vi "Set Header and Data.vi"(6 "Data Array":dbl[](array[numeric]), 8 "error in (no error)":errorcluster, 9 "Data & Time String":string, 10 "Header":string, 11 "Report.lvclass in":refnum<class "Wind Report.lvclass">) -> (0 "error out":errorcluster, 3 "Report.lvclass out":refnum<class "Wind Report.lvclass">)   [LabVIEW 2009, in "Wind Report.lvclass"]
doc: "This parent method sets object data and can operate on the child object.\n\nAAL 9/09"
uses:
  Wind Report.lvclass
  Wind Report.lvclass/Wind Report.ctl
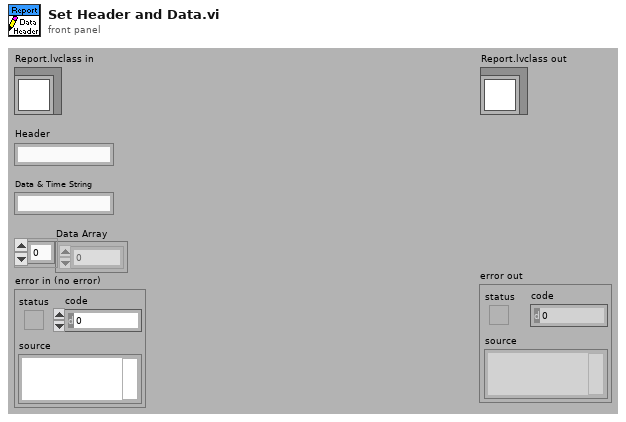
[diagram p1: front panel]
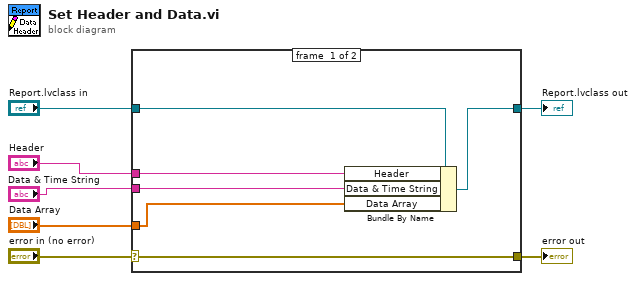
[diagram p0: block diagram]
diagram:
  n1 = case shown="No Error" "error in (no error)" {
    selector: "error in (no error)" -> [w13 w14]
    tunnel: [w13 w14] -> w6
    tunnel: [w11 w15] -> w4
    tunnel: "Report.lvclass in" -> [w12 w15]
    tunnel: "Header" -> [w10 _]
    tunnel: "Data & Time String" -> [w9 _]
    tunnel: "Data Array" -> [w8 _]
    frame #0 {
      n2 = Bundle By Name(cluster=w12, "Header"=w10, "Data & Time String"=w9, "Data Array"=w8) -> (w11:refnum<class "Wind Report.lvclass">)
    }
    frame #1 {
    }
  }
  "error out" <- w6
  "Report.lvclass out" <- w4
